vi "wait_stop_or_time.vi"(5 "ref_time_remain":refnum<vi>, 8 "ref_stop_internal":refnum<vi>, 10 "time_wait":i32, 11 "time0":timestamp) -> (0 "stop_out":bool)   [LabVIEW 2019]
panel:
  out "time_now":dbl
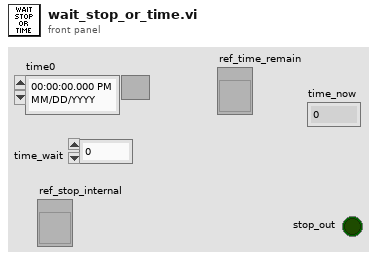
[diagram p1: front panel]
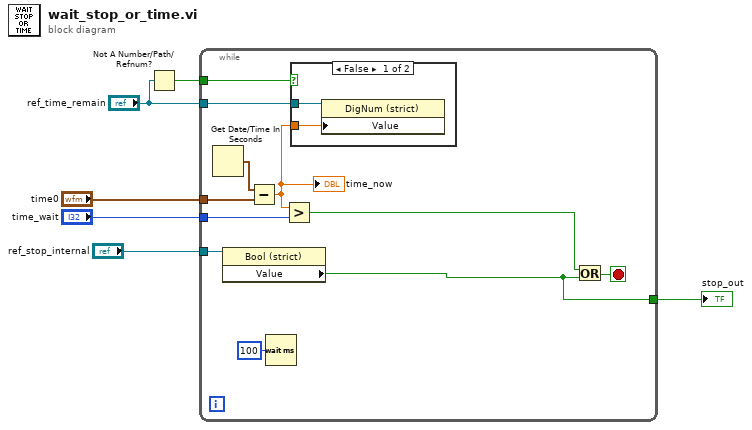
[diagram p0: block diagram]
diagram:
  n1 = Not A Number/Path/Refnum?(number/path/refnum="ref_time_remain") -> (NaN/Path/Refnum?=w1:bool)
  n2 = while {
    tunnel: "time0" -> [w15]
    tunnel: "time_wait" -> [w12]
    tunnel: "ref_stop_internal" -> [w11]
    tunnel: [w7] -> w3
    tunnel: "ref_time_remain" -> [w9]
    tunnel: w1 -> [w10]
    stop <- w13 stop-if-true
    n3 = Get Date/Time In Seconds() -> (seconds since 1Jan1904=w16:timestamp)
    n4 = property class="Bool (strict)"(reference=w11) -> ("Value"=w7:bool)  [unwired: 1 in, 2 out]
    n5 = Subtract(x=w16, y=w15) -> (x-y=w8:dbl)
    "time_now" <- w8
    n6 = Wait (ms)(milliseconds to wait=u32 100) -> ()  [unwired: 1 out]
    n7 = Greater?(x=w8, y=w12) -> (0:w14:bool)
    n8 = case shown="False" w10 {
      tunnel: w9 -> [w19 _]
      tunnel: w8 -> [w18 _]
      frame False {
        n9 = property on="Property Node" class="DigNum (strict)"(reference=w19, "Value"=w18) -> ()  [unwired: 1 in, 2 out]
      }
      frame True {
      }
    }
    n10 = Or(x=w14, y=w7) -> (x .or. y?=w13:bool)
  }
  "stop_out" <- w3
